vi "Parse State Queue++.vi"(0 "State Queue":string, 1 "Name(\"\" to use uuid)":string, 7 "Error In (no error)":errorcluster, 9 "Dequeue Timeout(0ms)":i32, 11 "Response Timeout(1000ms)":i32=1000) -> (4 "Remaining States":string, 6 "Current State":string, 8 "Arguments":string, 15 "From Who":string)   [LabVIEW 2020, in "JKI-State-Machine-Plus.lvlib"]
doc: "Parses the JKI State Machine state queue and returns the current state that will execute next with the associated arguments.\n\nFor instructions on how to use the JKI State Machine, examples and video tutorials, visit:\nhttp://jkisoft.com/state-machine/\n\n<B>Inputs:</B>\n <B>State Queue:</B> The entire state queue is wired to this input. This should come from the main JKI State Machine shift register.\n <B>Error In</B> The error cluster from the JKI State Machine is wired to this input. If an error occures and appears on this input, the current state output returns the \"Error Handler\" state.\n\n<B>Outputs:</B>\n <B>Remaining States:</B> Returns all the next states that should execute after the current state completes. These should be passed through the current state in the state machine. These can also be modified or augmented within the current state if necessary.\n <B>Current State:</B> Returns the current state that should execute next in the state machine. If an error is wired to the Error input then the current state output becomes \"Error Handler\".\n <B>Arguments:</B> Returns any argument(s) that may be used in the current state string. These arguments come after the \">>\" characters. <B>Note:</B> The arguments variable must not contain any unprintable characters like linefeed or carriage return.\n\n<B>State Syntax:</B>\nStateCategory: State >> Argument\nLine Terminator: Line feed\n <B>Example:</B>\nUI: Help >> About\n\nWhere \"UI\" is the state category\nWhere \"Help\" is the state\nWhere \"About\" is the argument\n <B>Other Examples:</B>\nApp Data: Initialize\nUI: Initialize\nHelp >> About\n\n<B>Commenting:</B>\nTo add a comment use \"//\" or \"#\" and all text to the right will be ignored\n <B>Commenting Example:</B>\nUI: Initialize // This initializes the UI\n# This whole line is a comment\n// Another comment line\n\nJKI State Machine™ 2018.0.7.45\nhttp://jki.net/state-machine/\nCopyright (C) 2005-2018, JKI <info@jki.net>\nALL RIGHTS RESERVED"
uses:
  JKI-State-Machine-Plus.lvlib
  _Cross JKI StateMachine State Data.ctl
  _Cross JKI StateMachine State Response.ctl
  <vilib>/addons/_JKI Toolkits/State Machine/_JKI_lib_State_Machine.llb/Add State(s) to Queue__JKI_lib_State_Machine.vi
  Build State String with Arguments Plus.vi
  _uuid.vi
  _JKISMQFGV.vi
  <vilib>/regexp/Match Regular Expression.xnode
panel:
  # "For instructions on how to use the JKI State Machine, examples and video tutorials, visit:\nhttp://jki.net/state-machine/\n\nJKI State Machine™\nhttp://jki.net/state-machine/\nCopyright (C) 2005-2017, JKI <info@jki.net>\nALL RIGHTS RESERVED"
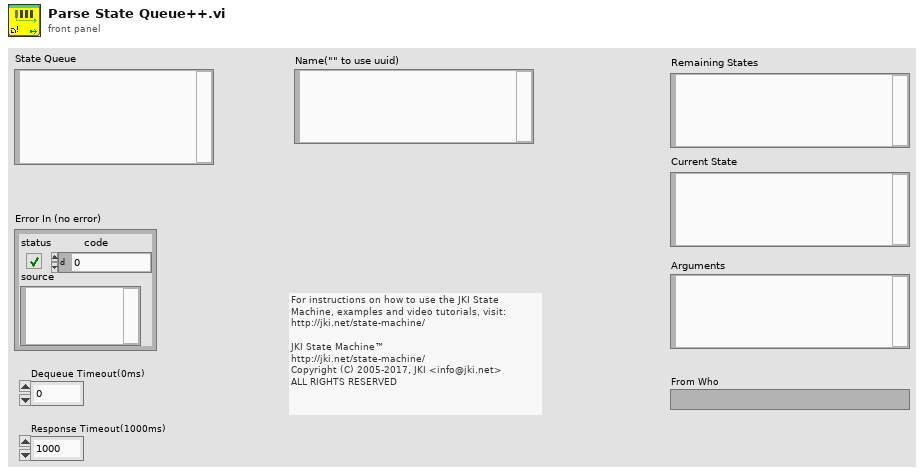
[diagram p1: front panel]
types:
  T1 = typedef "JKI-State-Machine-Plus.lvlib/_Cross JKI StateMachine State Data.ctl" = cluster{"state":string, "args":string, "source":string, "RespQ":refnum<queue>}
  T2 = typedef "JKI-State-Machine-Plus.lvlib/_Cross JKI StateMachine State Response.ctl" = cluster{"error":errorcluster}
  T3 = typedef "JKI-State-Machine-Plus.lvlib/_JKISMQ.ctl" = cluster{"Queue":refnum<queue>, "Locked Status":refnum<data-value>, "Stand Alone Mode":bool}
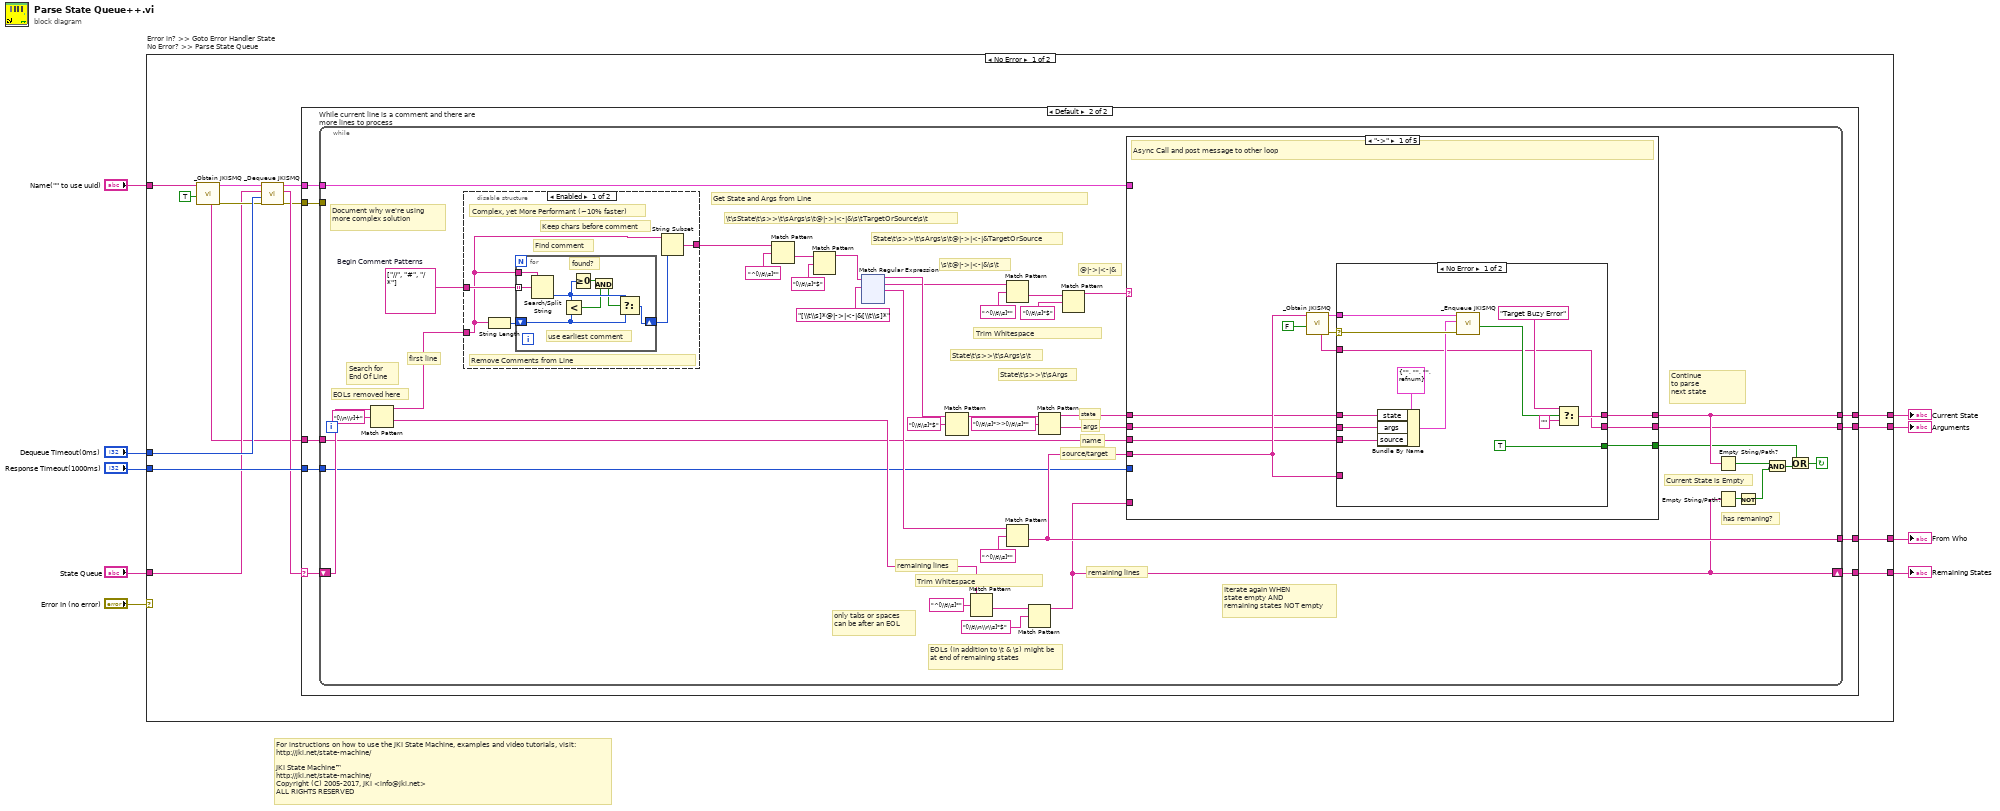
[diagram p0: block diagram]
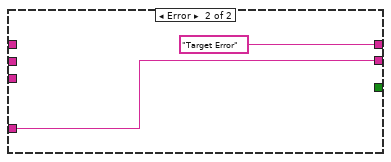
[diagram p3: hidden frame]
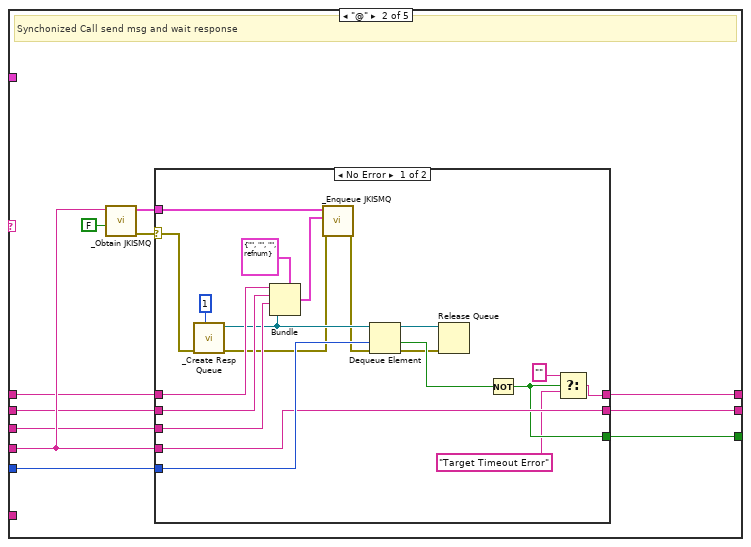
[diagram p4: hidden frame]
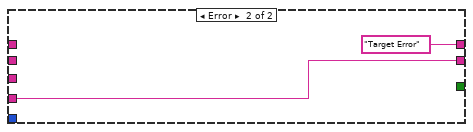
[diagram p5: hidden frame]
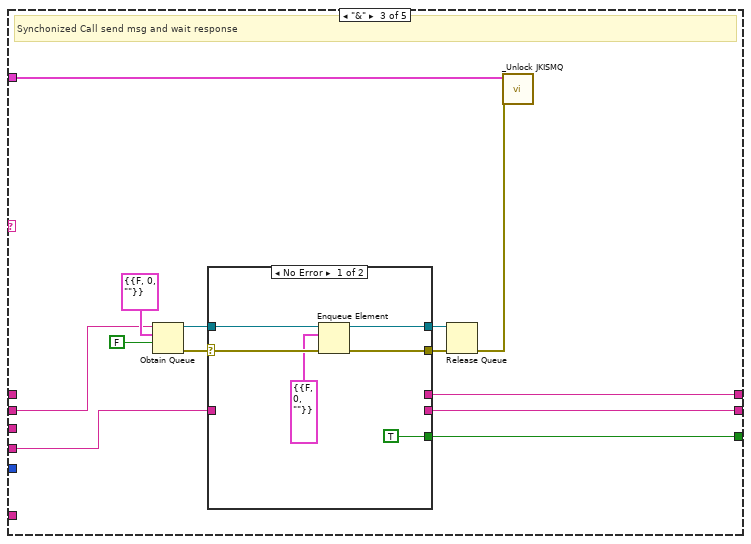
[diagram p6: hidden frame]
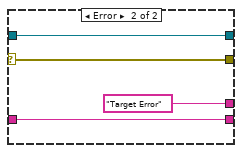
[diagram p7: hidden frame]
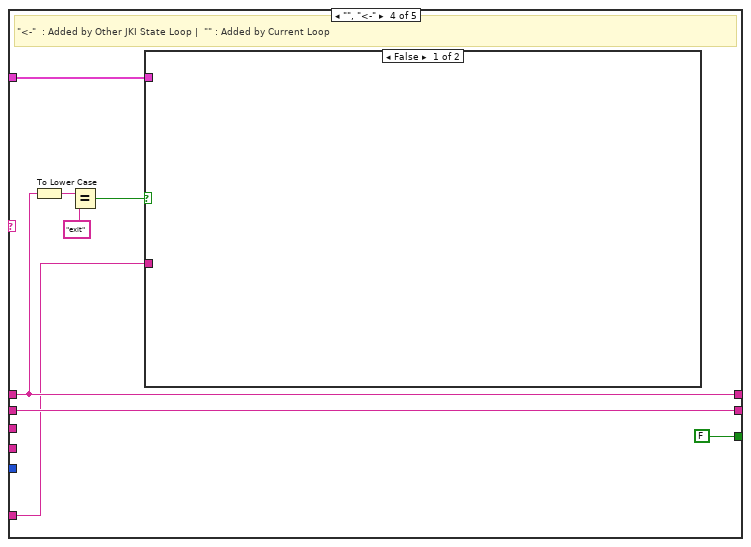
[diagram p8: hidden frame]
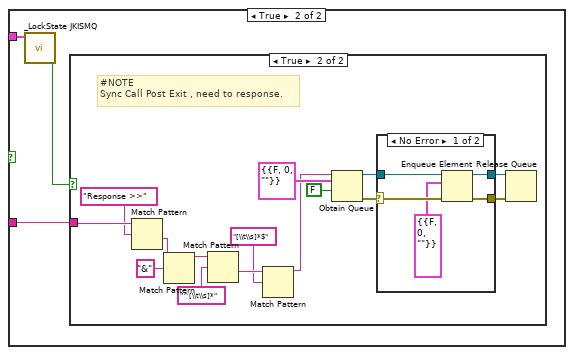
[diagram p9: hidden frame]
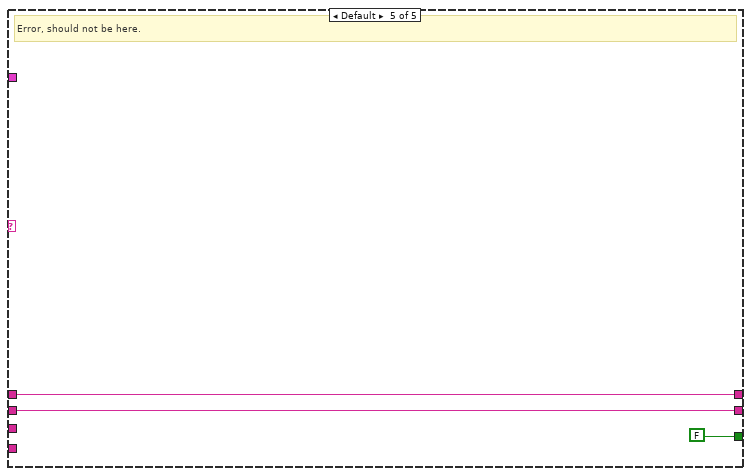
[diagram p12: hidden frame]
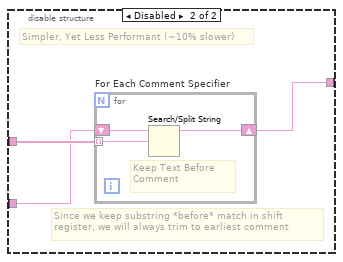
[diagram p13: hidden frame]
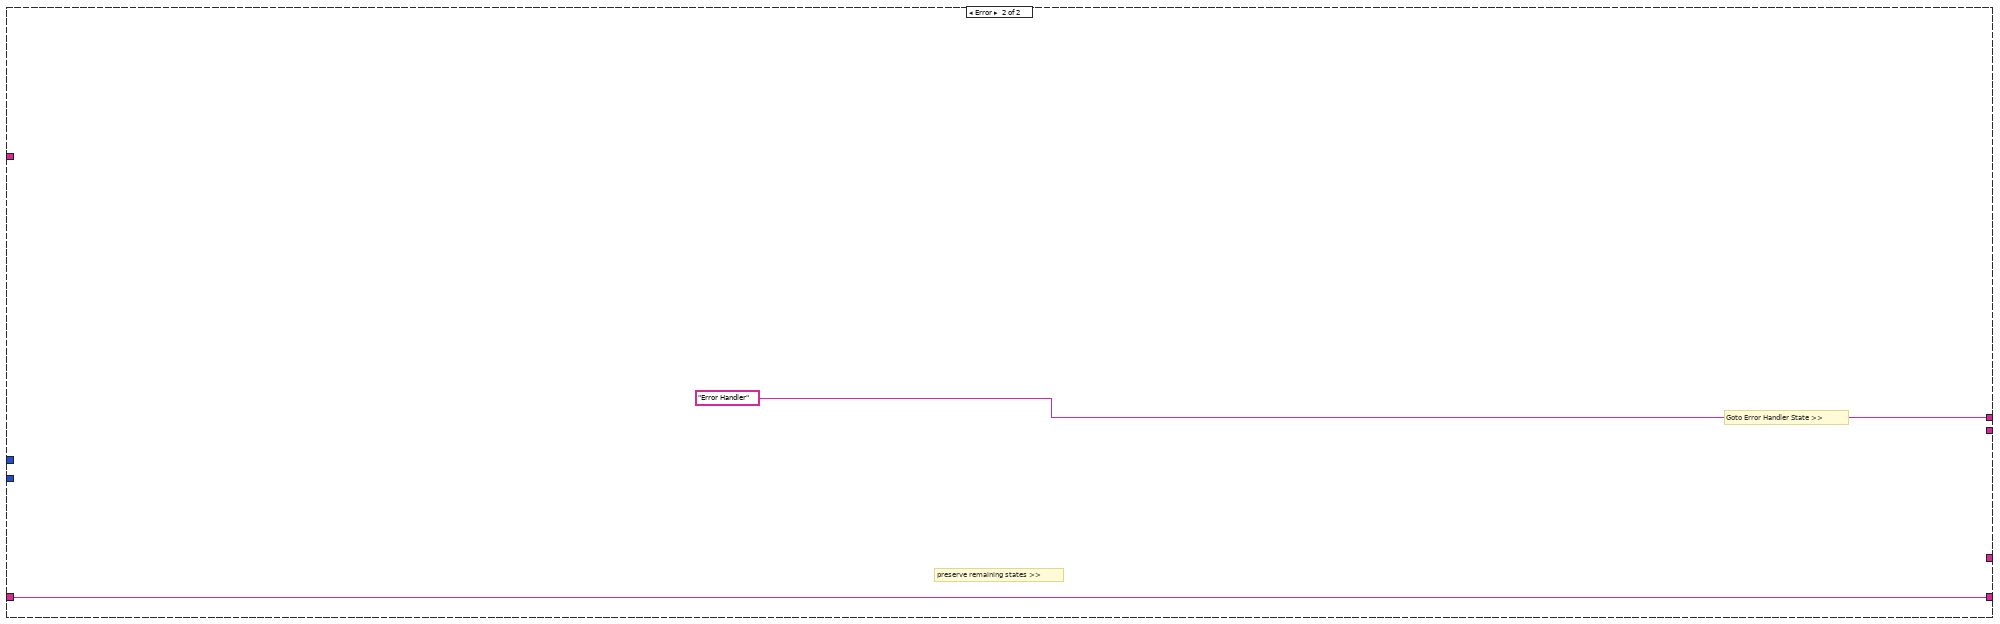
[diagram p14: hidden frame]
diagram:
  # "For instructions on how to use the JKI State Machine, examples and video tutorials, visit:\nhttp://jki.net/state-machine/\n\nJKI State Machine™\nhttp://jki.net/state-machine/\nCopyright (C) 2005-2017, JKI <info@jki.net>\nALL RIGHTS RESERVED"
  n1 = case "Error in? >> Goto Error Handler State\nNo Error? >> Parse State Queue" shown="No Error" "Error In (no error)" {
    tunnel: [w22 w326] -> w9
    tunnel: [w24 "Error Handler"] -> w7
    tunnel: [w23 _] -> w6
    tunnel: "State Queue" -> [w13 w326]
    tunnel: "Response Timeout(1000ms)" -> [w21 _]
    tunnel: "Name(\"\" to use uuid)" -> [w20 _]
    tunnel: [w19 _] -> w2
    tunnel: "Dequeue Timeout(0ms)" -> [w18 _]
    frame No Error {
      n2 = call "_Obtain JKISMQ.vi"("create if not found? (T)"=TRUE, "Name(\"\" to use uuid) in"=w20) -> ("Error out"=w15:errorcluster, "JKISMQ"=w17:T3, "Name"=w11:string)  [unwired: 6 in, 1 out]
      n3 = call "_Dequeue JKISMQ.vi"("Error in"=w15, "Dequeue Timeout(0ms)"=w18, "State(s) in (\"\")"=w13, "JKISMQ"=w17) -> ("Error out"=w10:errorcluster, "States Out"=w12:string, "JKISMQ"=w14:T3)  [unwired: 5 in]
      n4 = case shown="Default" w12 {
        selector: w12 -> [_ w27]
        tunnel: [_ w33] -> w24
        tunnel: [_ w32] -> w23
        tunnel: [_ w31] -> w22
        tunnel: w21 -> [_ w30]
        tunnel: [_ w29] -> w19
        tunnel: w11 -> [_ w28]
        tunnel: w14 -> [_ w26]
        tunnel: w10 -> [_ w25]
        frame "" {
          # "Do Nothing if Empty String"
          # "<< Wiring into the Case Selector is much more performant than using \"Empty String/Path?\" primitive"
        }
        frame Default {
          n5 = while "While current line is a comment and there are more lines to process" {
            tunnel: [w44] -> w33
            tunnel: [w43] -> w32
            shift-right: [w34] -> w31
            shift-left: w27 -> [w70]
            tunnel: w30 -> [w37]
            tunnel: w28 -> [w42]
            tunnel: [w41] -> w29
            tunnel: w26 -> [w35]
            tunnel: w25 -> [_]
            stop <- w40 continue-if-true
            w69 = string[] ["//", "#", "/*"]  # Begin Comment Patterns
            # "Continue\nto parse \nnext state"
            # "source/target"
            # "name"
            # "@|->|<-|&"
            # "\\s\\t@|->|<-|&\\s\\t"
            # "Trim Whitespace"
            # "State\\t\\s>>\\t\\sArgs"
            # "State\\t\\s>>\\t\\sArgs\\s\\t"
            # "Get State and Args from Line"
            # "State\\t\\s>>\\t\\sArgs\\s\\t@|->|<-|&TargetOrSource"
            # "\\t\\sState\\t\\s>>\\t\\sArgs\\s\\t@|->|<-|&\\s\\tTargetOrSource\\s\\t"
            # "remaining lines"
            # "EOLs (in addition to \\t & \\s) might be at end of remaining states"
            # "Document why we're using more complex solution"
            # "Trim Whitespace"
            # "EOLs removed here"
            # "only tabs or spaces can be after an EOL"
            # "Current State is Empty"
            # "has remaning?"
            # "remaining lines"
            # "first line"
            # "Search for End Of Line"
            # "Iterate again WHEN\nstate empty AND\nremaining states NOT empty"
            # "args"
            # "state"
            n6 = Match Pattern(string=w70, regular expression="[\\n\\r]+") -> (before substring=w67:string, after substring=w60:string)  [unwired: 1 in, 2 out]
            n7 = disable-structure "Diagram Disable Structure" shown="Enabled" {
              disable-tunnel: w69 -> [w310 w321]
              disable-tunnel: [w309 w320] -> w68
              disable-tunnel: w67 -> [w308 w319]
              frame Enabled {
                # "Remove Comments from Line"
                # "Complex, yet More Performant (~10% faster)"
                # "Keep chars before comment"
                # "Find comment"
                n8 = String Length(string=w308) -> (length=w307:i32)
                n9 = for {
                  tunnel: w310 -> [w315] mode=indexing
                  shift-right: [w317] -> w306
                  shift-left: w307 -> [w318]
                  tunnel: w308 -> [w316]
                  # "found?"
                  # "use earliest comment"
                  n10 = Search/Split String(string=w316, search string/char (-)=w315) -> (offset of match=w314:i32)  [unwired: 1 in, 2 out]
                  n11 = Less?(x=w314, y=w318) -> (x < y?=w312:bool)
                  n12 = Greater Or Equal To 0?(x=w314) -> (x >= 0?=w313:bool)
                  n13 = And(x=w313, y=w312) -> (x .and. y?=w311:bool)
                  n14 = Select(t=w314, s=w311, f=w318) -> (s? t:f=w317:i32)
                }
                n15 = String Subset(string=w308, length (rest)=w306) -> (substring=w309:string)  [unwired: 1 in]
              }
              frame Disabled {
                # "Since we keep substring *before* match in shift register, we will always trim to earliest comment"
                # "Simpler, Yet Less Performant (~10% slower)"
                n16 = for "For Each Comment Specifier" {
                  tunnel: w321 -> [w323] mode=indexing
                  shift-right: [w322] -> w320
                  shift-left: w319 -> [w324]
                  # "Keep Text Before Comment"
                  n17 = Search/Split String(string=w324, search string/char (-)=w323) -> (substring before match=w322:string)  [unwired: 1 in, 2 out]
                }
              }
            }
            n18 = Match Pattern(string=w68, regular expression="^[\\t\\s]*") -> (after substring=w58:string)  [unwired: 1 in, 3 out]
            n19 = Match Pattern(string=w58, regular expression="[\\t\\s]*$") -> (before substring=w36:string)  [unwired: 1 in, 3 out]
            n20 = xnode "Match Regular Expression"("input string"=w36, "regular expression"="[\\t\\s]*@|->|<-|&[\\t\\s]*") -> ("before match"=w55:string, "whole match"=w52:string, "after match"=w45:string)  [unwired: 4 in, 2 out]
            n21 = Match Pattern(string=w55, regular expression="[\\t\\s]*$") -> (before substring=w54:string)  [unwired: 1 in, 3 out]
            n22 = Match Pattern(string=w60, regular expression="^[\\t\\s]*") -> (after substring=w59:string)  [unwired: 1 in, 3 out]
            n23 = Match Pattern(string=w52, regular expression="^[\\t\\s]*") -> (after substring=w48:string)  [unwired: 1 in, 3 out]
            n24 = Match Pattern(string=w45, regular expression="^[\\t\\s]*") -> (after substring=w41:string)  [unwired: 1 in, 3 out]
            n25 = Match Pattern(string=w59, regular expression="[\\t\\n\\r\\s]*$") -> (before substring=w34:string)  [unwired: 1 in, 3 out]
            n26 = Match Pattern(string=w54, regular expression="[\\t\\s]*>>[\\t\\s]*") -> (before substring=w51:string, after substring=w50:string)  [unwired: 1 in, 2 out]
            n27 = Match Pattern(string=w48, regular expression="[\\t\\s]*$") -> (before substring=w47:string)  [unwired: 1 in, 3 out]
            n28 = case shown="\"->\"" w47 {
              tunnel: w51 -> [w77 w102 _ w161 w191]
              tunnel: w50 -> [w76 w101 w135 w163 w190]
              tunnel: [w83 w108 w144 w161 w191] -> w44
              tunnel: [w82 w107 w143 w163 w190] -> w43
              tunnel: w42 -> [w75 w100 _ _ _]
              tunnel: w41 -> [w80 w106 w136 _ _]
              tunnel: [w84 w109 w145 FALSE FALSE] -> w38
              tunnel: w37 -> [_ w110 _ _ _]
              tunnel: w35 -> [_ _ w134 w156 _]
              tunnel: w34 -> [_ _ _ w158 _]
              frame "->" {
                # "Async Call and post message to other loop"
                n29 = call "_Obtain JKISMQ.vi"("create if not found? (T)"=FALSE, "Name(\"\" to use uuid) in"=w80) -> ("Error out"=w78:errorcluster, "JKISMQ"=w79:T3, "Name"=w74:string)  [unwired: 6 in, 1 out]
                n30 = case shown="No Error" w78 {
                  selector: w78 -> [w96 _]
                  tunnel: w79 -> [w97 _]
                  tunnel: [TRUE _] -> w84
                  tunnel: [w86 "Target Error" ("before match")] -> w83
                  tunnel: [w85 w98] -> w82
                  tunnel: w80 -> [_ w98]
                  tunnel: w77 -> [w93 _]
                  tunnel: w76 -> [w92 _]
                  tunnel: w75 -> [w91 _]
                  tunnel: w74 -> [w85 _]
                  frame No Error {
                    n31 = Bundle By Name(cluster=T1 {"state"="", "args"="", "source"="", "RespQ"=refnum} ("Cross JKI State Machine State"), "state"=w93, "args"=w92, "source"=w91) -> (w90:T1)
                    n32 = call "_Enqueue JKISMQ.vi"("Error in"=w96, "Data"=w90, "JKISMQ"=w97) -> ("Target Buzy Error"=w87:bool)  [unwired: 6 in, 2 out]
                    n33 = Select(t="Target Buzy Error" ("f"), s=w87, f="" ("before match")) -> (s? t:f=w86:string)
                  }
                  frame Error {
                  }
                }
              }
              frame "@" {
                # "Synchonized Call send msg and wait response"
                n34 = call "_Obtain JKISMQ.vi"("create if not found? (T)"=FALSE, "Name(\"\" to use uuid) in"=w106) -> ("Error out"=w104:errorcluster, "JKISMQ"=w105:T3)  [unwired: 6 in, 2 out]
                n35 = case shown="No Error" w104 {
                  selector: w104 -> [w115 _]
                  tunnel: w110 -> [w129 _]
                  tunnel: w105 -> [w130 _]
                  tunnel: [w125 _] -> w109
                  tunnel: [w128 "Target Error" ("before match")] -> w108
                  tunnel: [w127 w131] -> w107
                  tunnel: w106 -> [w127 w131]
                  tunnel: w102 -> [w121 _]
                  tunnel: w101 -> [w120 _]
                  tunnel: w100 -> [w119 _]
                  frame No Error {
                    n36 = call "_Create Resp Queue.vi"("max queue size (-1, unlimited)"=1, "error in (no error)"=w115) -> ("error out"=w111:errorcluster, "queue out"=w116:refnum<queue>)  [unwired: 7 in, 1 out]
                    n37 = Bundle(cluster=T1 {"state"="", "args"="", "source"="", "RespQ"=refnum} ("Cross JKI State Machine State"), "state"=w121, "args"=w120, "source"=w119, "RespQ"=w116) -> (w117:T1)
                    n38 = call "_Enqueue JKISMQ.vi"("Error in"=w111, "Data"=w117, "JKISMQ"=w130) -> ("Error out"=w112:errorcluster)  [unwired: 6 in, 2 out]
                    n39 = Dequeue Element(queue=w116, timeout in ms (-1)=w129, error in (no error)=w112) -> (queue out=w114:refnum<queue>, timed out?=w126:bool, error out=w113:errorcluster)  [unwired: 1 out]
                    n40 = Release Queue(queue=w114, error in (no error)=w113) -> ()  [unwired: 1 in, 3 out]
                    n41 = Not(x=w126) -> (.not. x?=w125:bool)
                    n42 = Select(t="" ("f"), s=w125, f="Target Timeout Error" ("before match")) -> (s? t:f=w128:string)
                  }
                  frame Error {
                  }
                }
              }
              frame "&" {
                # "Synchonized Call send msg and wait response"
                n43 = Obtain Queue(name (unnamed)=w135, element data type=T2 {"error"={"status"=FALSE, "code"=0, "source"=""}} ("Cross JKI State Machine Response"), create if not found? (T)=FALSE) -> (queue out=w140:refnum<queue>, error out=w139:errorcluster)  [unwired: 2 in, 1 out]
                n44 = case shown="No Error" w139 {
                  selector: w139 -> [w149 w153]
                  tunnel: [TRUE _] -> w145
                  tunnel: [_ "Target Error" ("before match")] -> w144
                  tunnel: [_ w152] -> w143
                  tunnel: w140 -> [w151 w154]
                  tunnel: [w150 w154] -> w142
                  tunnel: [w148 w153] -> w141
                  tunnel: w136 -> [_ w152]
                  frame No Error {
                    n45 = Enqueue Element(queue=w151, element=T2 {"error"={"status"=FALSE, "code"=0, "source"=""}}, error in (no error)=w149) -> (queue out=w150:refnum<queue>, error out=w148:errorcluster)  [unwired: 1 in, 1 out]
                  }
                  frame Error {
                  }
                }
                n46 = Release Queue(queue=w142, error in (no error)=w141) -> (error out=w133:errorcluster)  [unwired: 1 in, 2 out]
                n47 = call "_Unlock JKISMQ.vi"("Error in"=w133, "JKISMQ"=w134) -> ()  [unwired: 8 in, 2 out]
              }
              frame "", "<-" {
                # "\"<-\"  : Added by Other JKI State Loop |  \"\" : Added by Current Loop"
                n48 = To Lower Case(string=w161) -> (all lower case string=w160:string)
                n49 = Equal?(x=w160, y="exit") -> (x = y?=w157:bool)
                n50 = case shown="False" w157 {
                  tunnel: w158 -> [_ w166]
                  tunnel: w156 -> [_ w165]
                  frame False {
                  }
                  frame True {
                    n51 = call "_LockState JKISMQ.vi"("JKISMQ"=w165) -> ("lock"=w164:bool)  [unwired: 8 in, 2 out]
                    n52 = case shown="True" w164 {
                      tunnel: w166 -> [_ w175]
                      frame False {
                      }
                      frame True {
                        # "#NOTE\nSync Call Post Exit , need to response."
                        n53 = Match Pattern(string=w175, regular expression="Response >>") -> (after substring=w172:string)  [unwired: 1 in, 3 out]
                        n54 = Match Pattern(string=w172, regular expression="&") -> (before substring=w168:string)  [unwired: 1 in, 3 out]
                        n55 = Match Pattern(string=w168, regular expression="^[\\t\\s]*") -> (after substring=w171:string)  [unwired: 1 in, 3 out]
                        n56 = Match Pattern(string=w171, regular expression="[\\t\\s]*$") -> (before substring=w167:string)  [unwired: 1 in, 3 out]
                        n57 = Obtain Queue(name (unnamed)=w167, element data type=T2 {"error"={"status"=FALSE, "code"=0, "source"=""}} ("Cross JKI State Machine Response"), create if not found? (T)=FALSE) -> (queue out=w180:refnum<queue>, error out=w181:errorcluster)  [unwired: 2 in, 1 out]
                        n58 = case shown="No Error" w181 {
                          selector: w181 -> [w184 w187]
                          tunnel: w180 -> [w186 w188]
                          tunnel: [w185 w188] -> w178
                          tunnel: [w183 w187] -> w179
                          frame No Error {
                            n59 = Enqueue Element(queue=w186, element=T2 {"error"={"status"=FALSE, "code"=0, "source"=""}}, error in (no error)=w184) -> (queue out=w185:refnum<queue>, error out=w183:errorcluster)  [unwired: 1 in, 1 out]
                          }
                          frame Error {
                          }
                        }
                        n60 = Release Queue(queue=w178, error in (no error)=w179) -> ()  [unwired: 1 in, 3 out]
                      }
                    }
                  }
                }
              }
              frame Default {
                # "Error, should not be here."
              }
            }
            n61 = Empty String/Path?(string/path=w44) -> (empty?=w73:bool)
            n62 = Empty String/Path?(string/path=w34) -> (empty?=w72:bool)
            n63 = Not(x=w72) -> (.not. x?=w66:bool)
            n64 = And(x=w73, y=w66) -> (x .and. y?=w39:bool)
            n65 = Or(x=w38, y=w39) -> (x .or. y?=w40:bool)
          }
        }
      }
    }
    frame Error {
      # "Goto Error Handler State >>"
      # "preserve remaining states >>"
    }
  }
  "Remaining States" <- w9
  "Arguments" <- w6
  "Current State" <- w7
  "From Who" <- w2
